vi "Indefinite Integral of Polynomial.vi"   [LabVIEW 2020, in "NI_AALPro.lvlib"]
doc: "Calculates the indefinite integral of <B>P(x)</B>. Wire data to the <B>P(x)</B> input to determine the polymorphic instance to use or manually select the instance."
uses:
  <vilib>/Analysis/NI_AALPro.lvlib
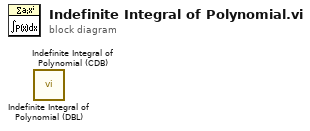
[diagram p0: block diagram]
diagram:
  n1 = call <vilib>:"Indefinite Integral of Polynomial (DBL).vi"() -> ()  [unwired: 10 in, 2 out]
  n2 = call <vilib>:"Indefinite Integral of Polynomial (CDB).vi"() -> ()  [unwired: 10 in, 2 out]
